vi "ds get case id.vi"(9 "dest_buffer_length":i32, 10 "BYTE_ARRAY":string, 11 "device_handle":u32) -> (1 "function return":i32, 2 "BYTE_ARRAY out":string, 3 "device_handle out":u32)   [LabVIEW 2019, in "apdm.lvlib"]
doc: "APDM_EXPORT int apdm_ds_get_case_id(apdm_device_handle_t device_handle, char *BYTE_ARRAY, const int dest_buffer_length);"
uses:
  apdm.lvlib
  Lee Lab/CP FES Walking 2018/Code/Working/LabVIEW/apdm.dll
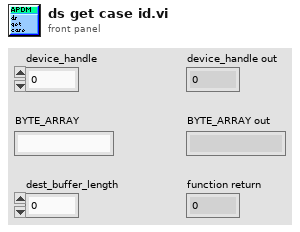
[diagram p1: front panel]
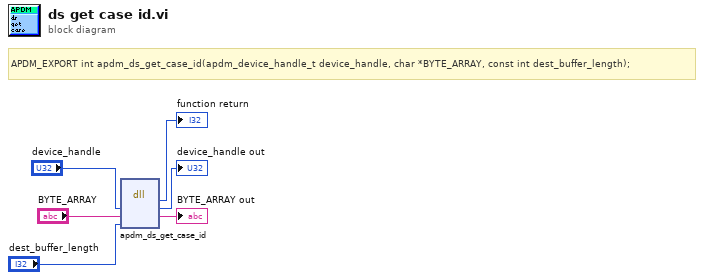
[diagram p0: block diagram]
diagram:
  # "APDM_EXPORT int apdm_ds_get_case_id(apdm_device_handle_t device_handle, char *BYTE_ARRAY, const int dest_buffer_length);"
  n1 = dll-call lib="C:/Users/jfalesi/Dropbox/Lee Lab/CP FES Walking 2018/Code/Working/LabVIEW/apdm.*" fn="apdm_ds_get_case_id"("device_handle"="device_handle", "BYTE_ARRAY"="BYTE_ARRAY", "dest_buffer_length"="dest_buffer_length") -> (→"function return":i32, "device_handle"=→"device_handle out":u32, "BYTE_ARRAY"=→"BYTE_ARRAY out":string)  [unwired: 4 in, 2 out]
